vi "testCheckSharedEnum.vi"(8 "error in (no error)":errorcluster) -> (0 "error out":errorcluster)   [LabVIEW 2018]
uses:
  SALTypeGenerator/Topic/Topic.lvclass
  <vilib>/addons/_JKI Toolkits/Caraya/classes/Assert/Assert Equal Value_Variant.vi
  <vilib>/addons/_JKI Toolkits/Caraya/classes/Test/Test.lvclass
  <vilib>/addons/_JKI Toolkits/Caraya/classes/Assert/Assert.lvclass
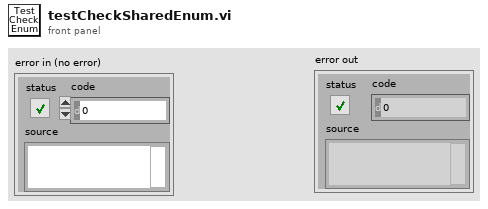
[diagram p1: front panel]
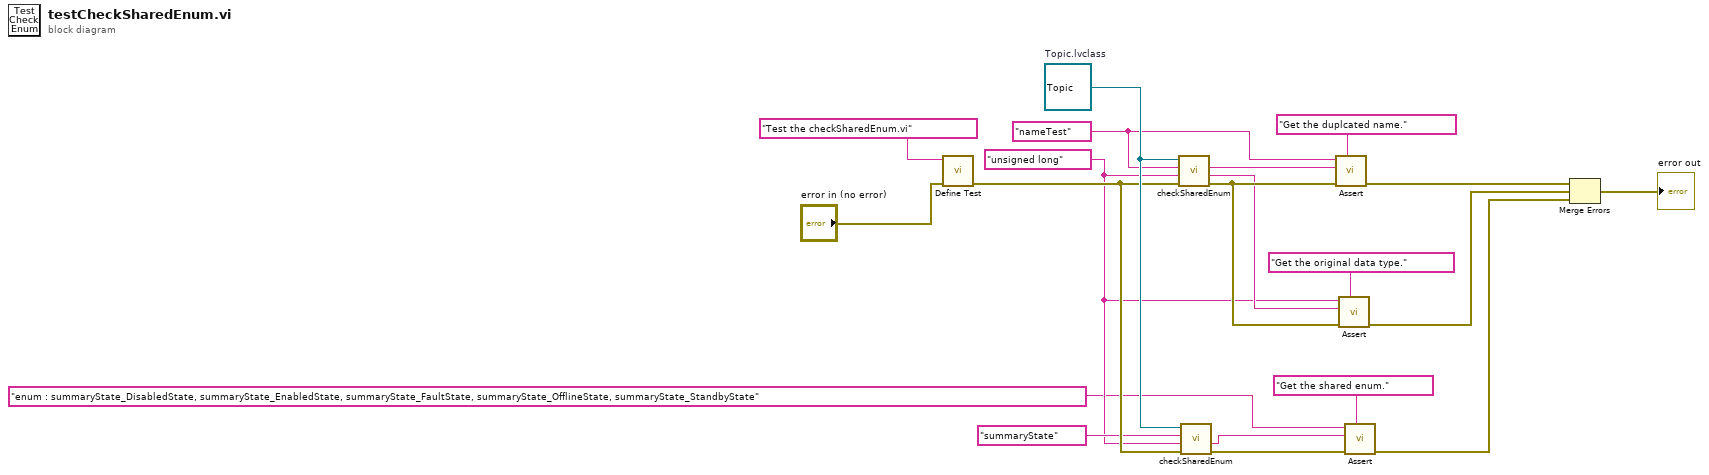
[diagram p0: block diagram]
diagram:
  w11 = "unsigned long"
  w12 = "nameTest"
  w18 = refnum<class "Topic.lvclass"> refnum  # Topic.lvclass
  n1 = call <vilib>:"Define Test.vi"("error in (no error)"="error in (no error)", "Label (VI Title)"="Test the checkSharedEnum.vi") -> ("error out"=w17:errorcluster)  [unwired: 9 in]
  n2 = call "checkSharedEnum.vi"("error in (no error)"=w17, "basicType"=w11, "name"=w12, "Topic in"=w18) -> ("error out"=w15:errorcluster, "basicTypeUpdated"=w14:string, "nameDup"=w13:string)  [unwired: 4 in, 1 out]
  n3 = call "checkSharedEnum.vi"("error in (no error)"=w17, "basicType"=w11, "name"="summaryState", "Topic in"=w18) -> ("error out"=w8:errorcluster, "basicTypeUpdated"=w7:string)  [unwired: 4 in, 2 out]
  n4 = call-poly <vilib>:"Assert.vi"("Label"="Get the duplcated name.", "error in (no error)"=w15, "Y"=w13, "X"=w12) -> ("error out"=w5:errorcluster)  [unwired: 7 in]
  n5 = call-poly <vilib>:"Assert.vi"("Label"="Get the original data type.", "error in (no error)"=w15, "Y"=w14, "X"=w11) -> ("error out"=w4:errorcluster)  [unwired: 7 in]
  n6 = call-poly <vilib>:"Assert.vi"("Label"="Get the shared enum.", "error in (no error)"=w8, "Y"=w7, "X"="enum : summaryState_DisabledState, summaryState_EnabledState, summaryState_FaultState, summaryState_OfflineState, summaryState_StandbyState") -> ("error out"=w3:errorcluster)  [unwired: 7 in]
  n7 = Merge Errors(w5, w4, w3) -> (→"error out":errorcluster)
